vi "AxxXY.vi"(4 "Y Tot":dbl, 5 "X Tot":dbl, 6 "Y Res":dbl, 7 "Y Center":dbl, 8 "X Res":dbl, 9 "X Center":dbl) -> (0 "YMIN":dbl, 1 "YMAX":dbl, 2 "XMIN":dbl, 3 "XMAX":dbl)   [LabVIEW 2019]
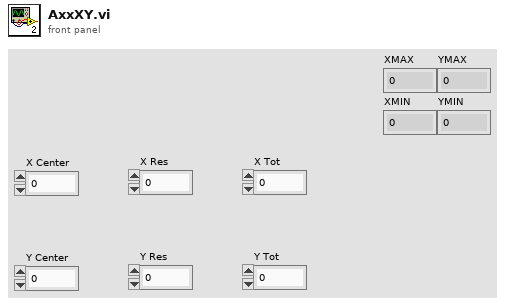
[diagram p1: front panel]
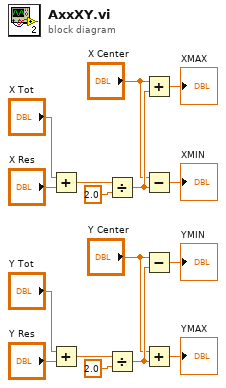
[diagram p0: block diagram]
diagram:
  n1 = Add(x="X Tot", y="X Res") -> (x+y=w14:dbl)
  n2 = Add(x="Y Tot", y="Y Res") -> (x+y=w6:dbl)
  n3 = Divide(x=w14, y=2.0) -> (x/y=w12:dbl)
  n4 = Divide(x=w6, y=2.0) -> (x/y=w8:dbl)
  n5 = Add(x="X Center", y=w12) -> (x+y=→"XMAX":dbl)
  n6 = Subtract(x="X Center", y=w12) -> (x-y=→"XMIN":dbl)
  n7 = Subtract(x="Y Center", y=w8) -> (x-y=→"YMIN":dbl)
  n8 = Add(x="Y Center", y=w8) -> (x+y=→"YMAX":dbl)
